vi "onHttpDelete.vi"(8 "error in":errorcluster, 10 "httpRequest":refnum<class "httpRequest.lvclass">, 11 "advanced-http-client in":refnum<class "advanced-http-client.lvclass">) -> (0 "error out":errorcluster, 2 "httpResponse":refnum<class "httpResponse.lvclass">, 3 "advanced-http-client out":refnum<class "advanced-http-client.lvclass">)   [LabVIEW 2020, in "HttpClient.NiAdvanced.lvlib" / "advanced-http-client.lvclass"]
uses:
  advanced-http-client.lvclass
  advanced-http-client.lvclass/advanced-http-client.ctl
  <vilib>/NI/Advanced HTTP Client/Session.lvclass
  http-client-pkg/httpRequest/httpRequest.lvclass
  http-client-pkg/httpResponse/httpResponse.lvclass
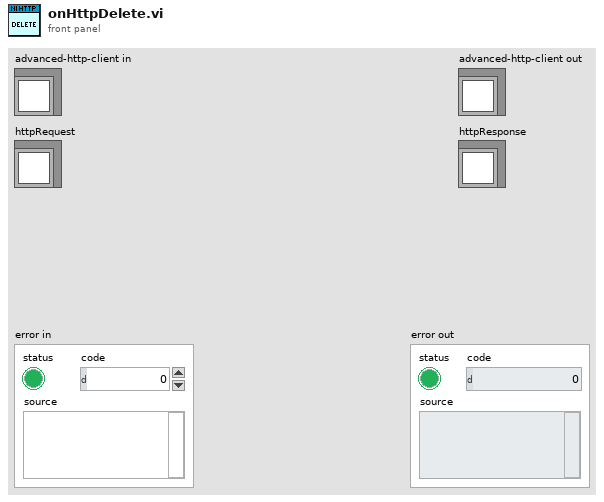
[diagram p1: front panel]
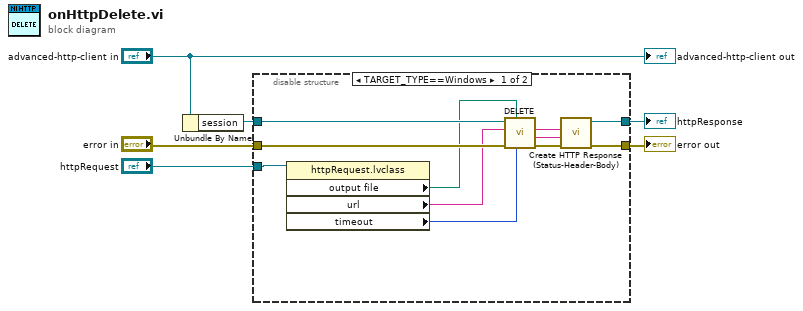
[diagram p0: block diagram]
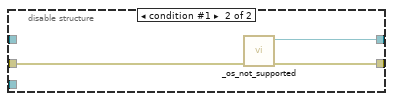
[diagram p2: hidden frame]
diagram:
  n1 = Unbundle By Name("advanced-http-client in") -> ("session"=w5:refnum<class "Session.lvclass">)
  n2 = disable-structure shown="TARGET_TYPE==Windows" {
    disable-tunnel: w5 -> [w17 _]
    disable-tunnel: "error in" -> [w16 w20]
    disable-tunnel: [w7 w19] -> w3
    disable-tunnel: "httpRequest" -> [w15 _]
    disable-tunnel: [w9 w18] -> w1
    frame condition #0 (active) {
      n3 = property class="httpRequest.lvclass"(reference=w15) -> ("output file"=w13:path, "url"=w14:string, "timeout"=w12:i32)  [unwired: 1 in, 2 out]
      n4 = call <vilib>:"DELETE.vi"("timeout"=w12, "output file"=w13, "error in"=w16, "url"=w14, "session in"=w17) -> ("error out"=w8:errorcluster, "body"=w11:string, "headers"=w10:string)  [unwired: 2 in, 2 out]
      n5 = call "Create HTTP Response (Status-Header-Body).vi"("error in"=w8, "body"=w11, "Headers w/ status line(s)"=w10) -> ("error out"=w7:errorcluster, "httpResponse out"=w9:refnum<class "httpResponse.lvclass">)  [unwired: 7 in]
    }
    frame condition #1 {
      n6 = call "_os_not_supported.vi"("error in (no error)"=w20) -> ("error out"=w19:errorcluster, "httpResponse"=w18:refnum<class "httpResponse.lvclass">)  [unwired: 9 in]
    }
  }
  "error out" <- w3
  "httpResponse" <- w1
  "advanced-http-client out" <- "advanced-http-client in"
